vi "room put.vi"(7 "side?":bool, 8 "error in (no error)":errorcluster, 9 "Position in":T1, 10 "register address":i32, 11 "put layer":i32) -> (0 "error out":errorcluster, 1 "Position out":T1)   [LabVIEW 2019]
uses:
  subVI/move/position cluster.ctl
  servo state.ctl
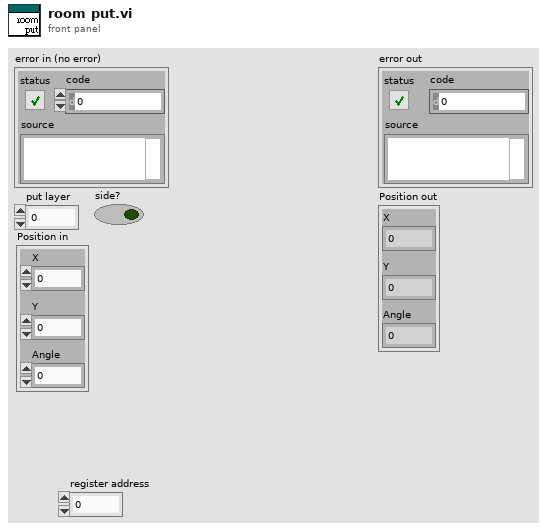
[diagram p1: front panel]
types:
  T1 = typedef "position cluster.ctl" = cluster{"X":dbl, "Y":dbl, "Angle":dbl}
  T2 = typedef "servo state.ctl" = enum16{"catch", "cam-1", "put", "side", "center", "side-2", "put-2"}
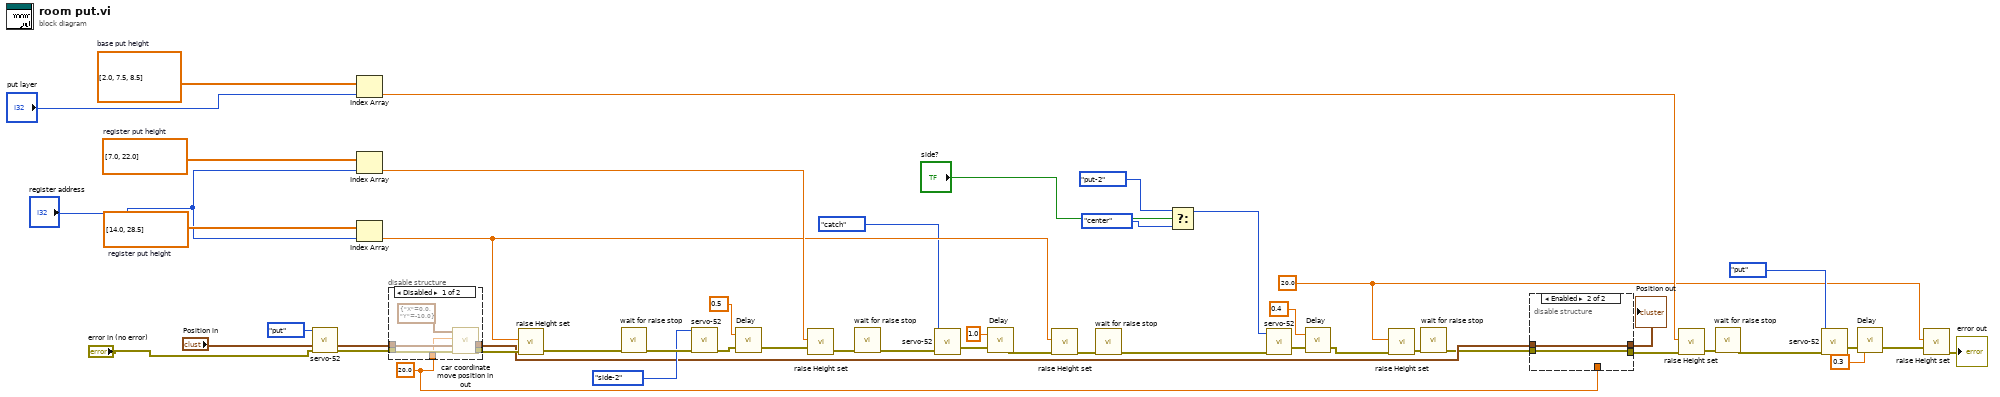
[diagram p0: block diagram]
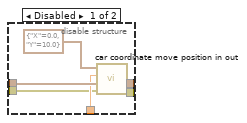
[diagram p3: hidden frame]
diagram:
  w21 = 20.0 ("Height_cm")
  w31 = 20.0 ("speed")
  w36 = dbl[] [2.0, 7.5, 8.5]  # base put height
  w47 = dbl[] [7.0, 22.0]  # register put height
  w48 = dbl[] [14.0, 28.5]  # register put height
  n1 = call "servo-52.vi"("error in (no error)"="error in (no error)", "Enum"=servo_state."put") -> ("error out"=w8:errorcluster)  [unwired: 9 in]
  n2 = Index Array(array=w36, index="put layer") -> (element=w25:dbl)
  n3 = Index Array(array=w47, index="register address") -> (element=w40:dbl)
  n4 = Index Array(array=w48, index="register address") -> (element=w38:dbl)
  n5 = disable-structure shown="Disabled" {
    disable-tunnel: [w54 w55] -> w34
    disable-tunnel: w8 -> [w53 w55]
    disable-tunnel: "Position in" -> [w52 w56]
    disable-tunnel: [w50 w56] -> w32
    disable-tunnel: w31 -> [w49 _]
    frame Disabled {
      n6 = call "car coordinate move position in out.vi"("error in (no error)"=w53, "Position in"=w52, "speed"=w49, "move"=cluster{"X":dbl, "Y":dbl} {"X"=0.0, "Y"=-10.0}) -> ("error out"=w54:errorcluster, "Position out"=w50:T1)  [unwired: 6 in]
    }
    frame Enabled {
    }
  }
  n7 = call "raise Height set.vi"("error in (no error)"=w34, "Height_cm"=w38) -> ("error out"=w45:errorcluster)  [unwired: 9 in]
  n8 = call "wait for raise stop.vi"("Error In"=w45) -> ("Error Out"=w44:errorcluster)  [unwired: 10 in]
  n9 = call "servo-52.vi"("error in (no error)"=w44, "Enum"=servo_state."side-2") -> ("error out"=w42:errorcluster)  [unwired: 9 in]
  n10 = call "Delay.vi"("error in (no error)"=w42, "Delay Time (s)"=0.5) -> ("error out"=w41:errorcluster)  [unwired: 1 in]
  n11 = call "raise Height set.vi"("error in (no error)"=w41, "Height_cm"=w40) -> ("error out"=w39:errorcluster)  [unwired: 9 in]
  n12 = call "wait for raise stop.vi"("Error In"=w39) -> ("Error Out"=w16:errorcluster)  [unwired: 10 in]
  n13 = call "servo-52.vi"("error in (no error)"=w16, "Enum"=servo_state."catch") -> ("error out"=w13:errorcluster)  [unwired: 9 in]
  n14 = call "Delay.vi"("error in (no error)"=w13, "Delay Time (s)"=1.0) -> ("error out"=w14:errorcluster)  [unwired: 1 in]
  n15 = call "raise Height set.vi"("error in (no error)"=w14, "Height_cm"=w38) -> ("error out"=w15:errorcluster)  [unwired: 9 in]
  n16 = call "wait for raise stop.vi"("Error In"=w15) -> ("Error Out"=w5:errorcluster)  [unwired: 10 in]
  n17 = Select(t=servo_state."put-2", s="side?", f=servo_state."center" ("Enum")) -> (s? t:f=w12:T2)
  n18 = call "servo-52.vi"("error in (no error)"=w5, "Enum"=w12) -> ("error out"=w30:errorcluster)  [unwired: 9 in]
  n19 = call "Delay.vi"("error in (no error)"=w30, "Delay Time (s)"=0.4) -> ("error out"=w29:errorcluster)  [unwired: 1 in]
  n20 = call "raise Height set.vi"("error in (no error)"=w29, "Height_cm"=w21) -> ("error out"=w28:errorcluster)  [unwired: 9 in]
  n21 = call "wait for raise stop.vi"("Error In"=w28) -> ("Error Out"=w27:errorcluster)  [unwired: 10 in]
  n22 = disable-structure shown="Enabled" {
    disable-tunnel: w32 -> [w62 w64]
    disable-tunnel: w31 -> [w61 _]
    disable-tunnel: w27 -> [w59 w63]
    disable-tunnel: [w58 w63] -> w26
    disable-tunnel: [w57 w64] -> w17
    frame Disabled {
      n23 = call "car coordinate move position in out.vi"("error in (no error)"=w59, "Position in"=w62, "speed"=w61, "move"=cluster{"X":dbl, "Y":dbl} {"X"=0.0, "Y"=10.0}) -> ("error out"=w58:errorcluster, "Position out"=w57:T1)  [unwired: 6 in]
    }
    frame Enabled {
    }
  }
  "Position out" <- w17
  n24 = call "raise Height set.vi"("error in (no error)"=w26, "Height_cm"=w25) -> ("error out"=w24:errorcluster)  [unwired: 9 in]
  n25 = call "wait for raise stop.vi"("Error In"=w24) -> ("Error Out"=w23:errorcluster)  [unwired: 10 in]
  n26 = call "servo-52.vi"("error in (no error)"=w23, "Enum"=servo_state."put") -> ("error out"=w20:errorcluster)  [unwired: 9 in]
  n27 = call "Delay.vi"("error in (no error)"=w20, "Delay Time (s)"=0.3) -> ("error out"=w19:errorcluster)  [unwired: 1 in]
  n28 = call "raise Height set.vi"("error in (no error)"=w19, "Height_cm"=w21) -> ("error out"=→"error out":errorcluster)  [unwired: 9 in]
